vi "GlobalDashboard.vi"() -> ()   [LabVIEW 2023]
doc: "Contains any of the global variables used by the Dashboard."
panel:
  out "Code_is_Running":bool
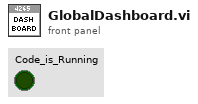
[diagram p1: front panel]
diagram:
